vi "generic_read_config_file.vi"(8 "error in (no error)":errorcluster, 10 "config cluster variant in (data type)":variant, 11 "GenericPlugin in":refnum<class "GenericComponent.lvclass">) -> (0 "error out":errorcluster, 2 "config cluster variant out (populated":variant, 3 "GenericPlugin out":refnum<class "GenericComponent.lvclass">)   [LabVIEW 2010, in "GenericComponent.lvclass"]
uses:
  GenericComponent.lvclass
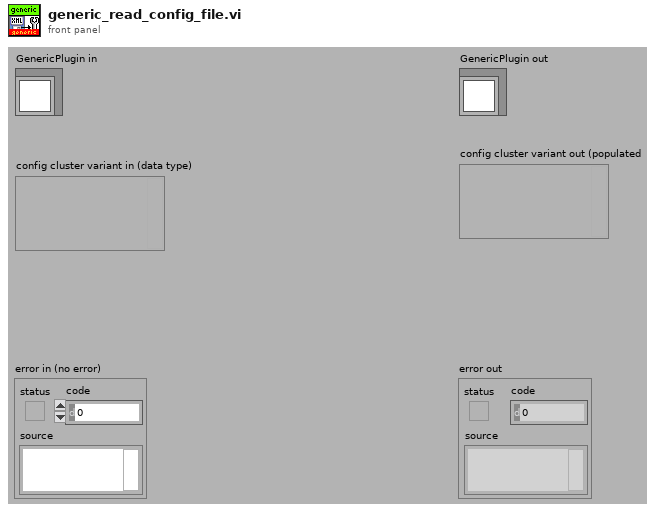
[diagram p1: front panel]
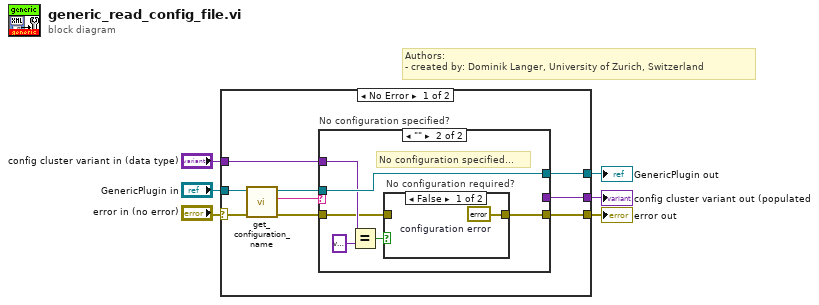
[diagram p0: block diagram]
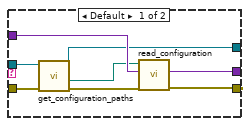
[diagram p2: hidden frame]
diagram:
  # "Authors: \n- created by: Dominik Langer, University of Zurich, Switzerland"
  n1 = case shown="No Error" "error in (no error)" {
    selector: "error in (no error)" -> [w9 w34]
    tunnel: [w13 w34] -> w6
    tunnel: [w12 w33] -> w4
    tunnel: "GenericPlugin in" -> [w11 w33]
    tunnel: "config cluster variant in (data type)" -> [w15 w32]
    tunnel: [w14 w32] -> w2
    frame No Error {
      n2 = call "get_configuration_name.vi"("error in (no error)"=w9, "GenericPlugin.lvclass in"=w11) -> ("error out"=w8:errorcluster, "configuration name"=w7:string, "GenericPlugin.lvclass out"=w10:refnum<class "GenericComponent.lvclass">)  [unwired: 7 out]
      n3 = case "No configuration specified?" shown="\"\"" w7 {
        tunnel: w15 -> [w23 w27]
        tunnel: [w22 _] -> w14
        tunnel: [w21 w28] -> w13
        tunnel: [w18 w29] -> w12
        tunnel: w10 -> [w17 w29]
        tunnel: w8 -> [w16 w24]
        frame Default {
          n4 = call-dynamic "get_configuration_paths.vi"("error in (no error)"=w16, "GenericComponent in"=w17) -> ("error out"=w19:errorcluster, "configuration file path"=w20:path, "GenericComponent out"=w18:refnum<class "GenericComponent.lvclass">)  [unwired: 2 in, 5 out]
          n5 = call "read_configuration.vi"("error in (no error)"=w19, "config cluster variant in (data type)"=w23, "path"=w20) -> ("error out"=w21:errorcluster, "config cluster variant out (populated"=w22:variant)  [unwired: 4 in, 3 out]
        }
        frame "" {
          # "No configuration specified..."
          n6 = Equal?(x=w27, y=variant ("x")) -> (x = y?=w25:bool)
          n7 = case "No configuration required?" shown="False" w25 {
            tunnel: [w30 w31] -> w28
            tunnel: w24 -> [_ w31]
            frame False {
              w30 = errorcluster {"status"=TRUE, "code"=-100, "source"="Configuration was empty"}  # configuration error
            }
            frame True {
            }
          }
        }
      }
    }
    frame Error {
    }
  }
  "error out" <- w6
  "GenericPlugin out" <- w4
  "config cluster variant out (populated" <- w2
